vi "parcour_fahren.vi"() -> ()   [LabVIEW 2019]
uses:
  <vilib>/Analysis/_algsub.llb/Vector Norm Type.ctl
  <vilib>/Analysis/baseanly.llb/A x Vector.vi
  <vilib>/Analysis/_algsub.llb/Real Vector Norm.vi
  parcour_liste/parcour_Liste.lvclass
  <vilib>/Analysis/NI_AALPro.lvlib
  <vilib>/Analysis/NI_AALBase.lvlib
panel:
  in  "gain Lenkung":dbl=0.5
  in  "Startkoord":dbl[](array[numeric])=[0.0, 0.0, 0.0]
  in  "v":dbl=20.0
  in  "Ts":dbl=0.02
  out "Sensorwert c":dbl format="%_4g"
  out "Position":dbl[](array[numeric])=[13.46599999999989, 0.0, 0.0] format="%_3g"
  out "XY Graph":cluster{"x":dbl[], "y":dbl[]}[](graph)=[{"x"=[0.0, 200.0], "y"=[0.0, 0.0]}, {"x"=[260.0, 259.2613004357083, 257.0633909777092, 253.4603914513021, 248.54101966249686, 242.42640687119285, 235.2671151375484, 227.2394299843728, 218.54101966249684, 209.38606790241386, 200.0], "y"=[60.0, 50.613932097586144, 41.45898033750316, 32.760570015627195, 24.732884862451613, 17.573593128807154, 11.45898033750315, 6.5396085486979345, 2.9366090222907886, 0.7386995642917356, 0.0]}, {"x"=[260.0, 259.5075336238055, 258.04226065180615, 255.64026096753472, 252.3606797749979, 248.2842712474619, 243.51141009169893, 238.15961998958187, 232.3606797749979, 226.25737860160925, 220.0], "y"=[60.0, 66.25737860160923, 72.36067977499789, 78.15961998958187, 83.51141009169893, 88.2842712474619, 92.36067977499789, 95.64026096753472, 98.04226065180615, 99.50753362380551, 100.0]}, {"x"=[0.0, 220.0], "y"=[100.0, 100.0]}, {"x"=[-40.0, -39.507533623805514, -38.04226065180614, -35.640260967534715, -32.3606797749979, -28.284271247461902, -23.511410091698927, -18.159619989581874, -12.360679774997898, -6.257378601609237, -2.4492935982947065e-15], "y"=[60.0, 66.25737860160923, 72.36067977499789, 78.15961998958187, 83.51141009169893, 88.2842712474619, 92.36067977499789, 95.64026096753472, 98.04226065180615, 99.50753362380551, 100.0]}, {"x"=[-40.0, -40.0], "y"=[60.0, 40.0]}, {"x"=[-40.0, -39.507533623805514, -38.04226065180614, -35.640260967534715, -32.3606797749979, -28.284271247461902, -23.511410091698927, -18.159619989581874, -12.360679774997898, -6.257378601609237, -2.4492935982947065e-15], "y"=[40.0, 33.74262139839077, 27.639320225002102, 21.84038001041813, 16.488589908301073, 11.715728752538102, 7.639320225002102, 4.359739032465285, 1.9577393481938614, 0.49246637619448563, 0.0]}, {"x"=[13.46599999999989, 35.46599999999989, 35.46599999999989, 13.46599999999989, 13.46599999999989], "y"=[7.0, 7.0, -7.0, -7.0, 7.0]}, {"x"=[10.46599999999989, 16.465999999999887, 16.465999999999887, 10.46599999999989, 10.46599999999989], "y"=[8.5, 8.5, 7.5, 7.5, 8.5]}, {"x"=[10.46599999999989, 16.465999999999887, 16.465999999999887, 10.46599999999989, 10.46599999999989], "y"=[-7.5, -7.5, -8.5, -8.5, -7.5]}, {"x"=[32.46599999999989, 38.46599999999989, 38.46599999999989, 32.46599999999989, 32.46599999999989], "y"=[8.5, 8.5, 7.5, 7.5, 8.5]}, {"x"=[32.46599999999989, 38.46599999999989, 38.46599999999989, 32.46599999999989, 32.46599999999989], "y"=[-7.5, -7.5, -8.5, -8.5, -7.5]}, {"x"=[36.46599999999989, 36.46599999999989, 36.46599999999989, 36.46599999999989, 36.46599999999989], "y"=[6.0, 0.0, -6.0, -6.0, -6.0]}]
  out "Lenkwinkel [rad]":dbl
  in  "stop":bool
  in  "milliseconds to wait":u32=10
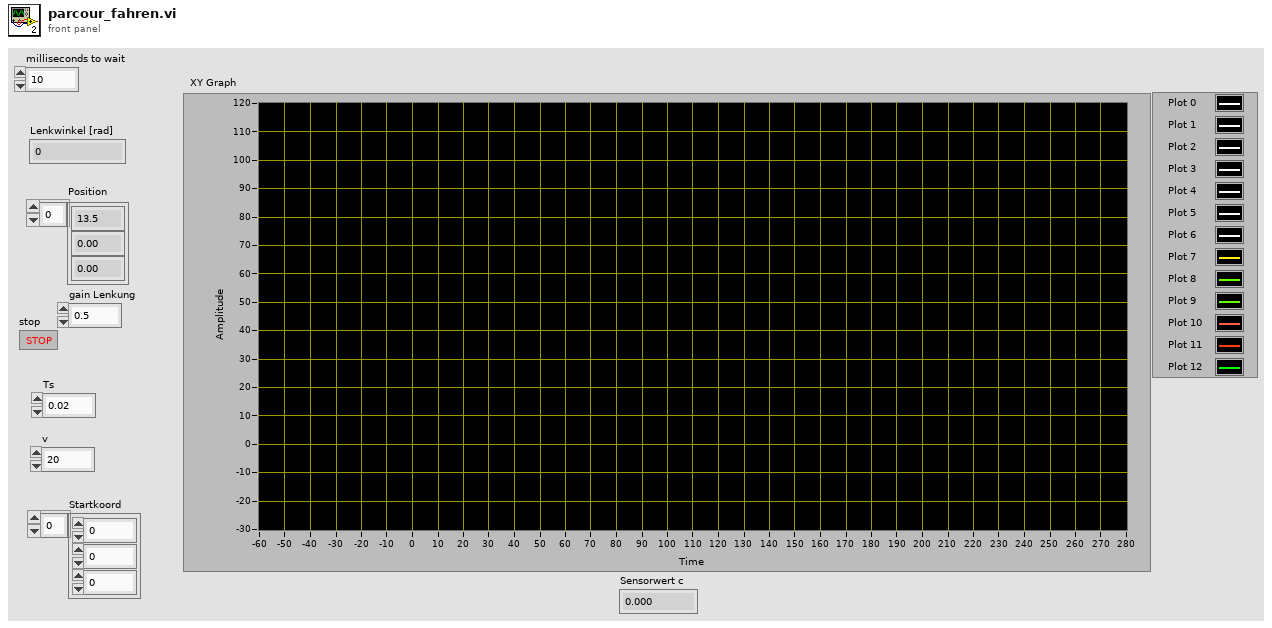
[diagram p1: front panel]
types:
  T1 = typedef "NI_Matrix.lvlib/RealMatrix.ctl" = dbl[][]
  T2 = typedef "NI_AALPro.lvlib/Vector Norm Type.ctl" = u16
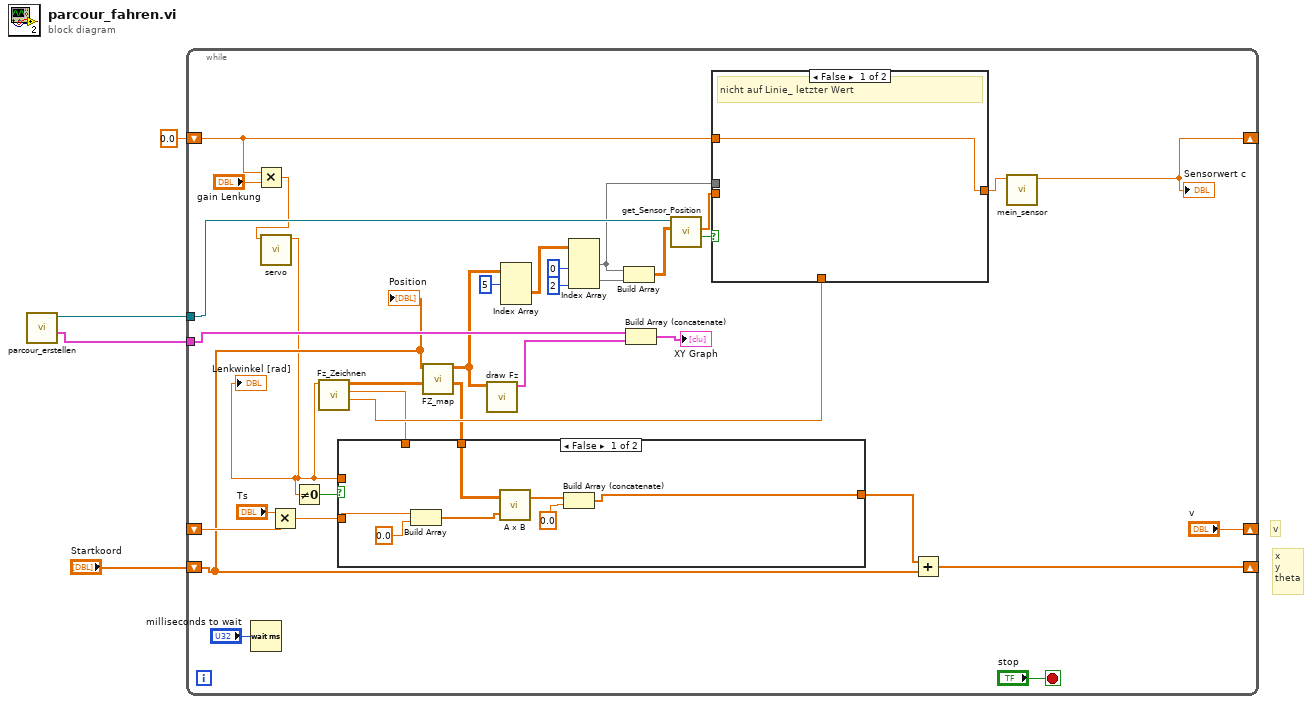
[diagram p0: block diagram]
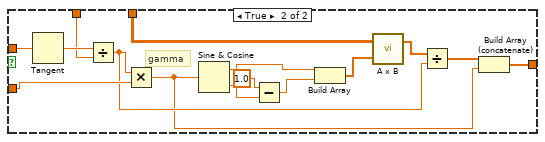
[diagram p2: hidden frame]
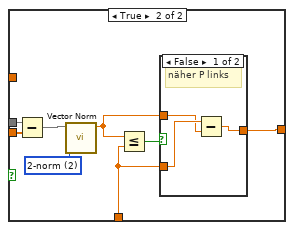
[diagram p3: hidden frame]
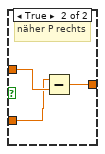
[diagram p4: hidden frame]
diagram:
  # "x\ny\ntheta"
  # "v"
  n1 = call "parcour_erstellen.vi"() -> ("XY_Parcout"=w3:cluster{"x":dbl[], "y":dbl[]}[], "parcour_Liste out"=w4:refnum<class "parcour_Liste.lvclass">)  [unwired: 10 in]
  n2 = while {
    tunnel: w4 -> [w25]
    tunnel: w3 -> [w36]
    shift-right: [w5] -> _
    shift-left: 0.0 -> [w9]
    shift-right: ["v"] -> _
    shift-left: _ -> [w16]
    shift-right: [w12] -> _
    shift-left: "Startkoord" -> [w11]
    stop <- "stop" stop-if-true
    n3 = Wait (ms)(milliseconds to wait="milliseconds to wait") -> ()  [unwired: 1 out]
    n4 = Multiply(x=w9, y="gain Lenkung") -> (x*y=w7:dbl)
    n5 = call "servo.vi"("Winkel soll"=w7) -> ("Winkel ist"=w6:dbl)  [unwired: 10 in]
    "Lenkwinkel [rad]" <- w6
    n6 = Multiply(x="Ts", y=w16) -> (x*y=w15:dbl)
    n7 = Not Equal To 0?(x=w6) -> (x != 0?=w10:bool)
    n8 = call "Fz_Zeichnen.vi"("Lenkwinkel [rad]"=w6) -> ("Breite Sensor/2 [cm] out"=w22:dbl, "Achsabstand [cm] out"=w18:dbl, "Fz"=w35:dbl[][][])  [unwired: 8 in]
    n9 = call "FZ_map.vi"("Fz"=w35, "Position"=w11) -> ("Rot(theta)"=w14:dbl[][], "FZ-mapped"=w32:dbl[][][])  [unwired: 8 in]
    n10 = case shown="False" w10 {
      tunnel: w6 -> [_ w60]
      tunnel: w18 -> [_ w58]
      tunnel: w15 -> [w45 w57]
      tunnel: w14 -> [w43 w51]
      tunnel: [w39 w46] -> w13
      frame False {
        n11 = Build Array(w45, 0.0 ("element")) -> (w42:dbl[])
        n12 = call-poly <vilib>:"A x B.vi"("Vector"=w42, "A"=w43) -> ("A x Vector"=w41:dbl[])  [unwired: 1 out]
        n13 = Build Array (concatenate)(w41, 0.0 ("element")) -> (w39:dbl[])
      }
      frame True {
        # "gamma"
        n14 = Tangent(1:w60) -> (0:w59:dbl)
        n15 = Divide(x=w59, y=w58) -> (x/y=w49:dbl)
        n16 = Multiply(x=w49, y=w57) -> (x*y=w47:dbl)
        n17 = Sine & Cosine(0:w47) -> (1:w53:dbl, 2:w56:dbl)
        n18 = Subtract(x=1.0, y=w56) -> (x-y=w54:dbl)
        n19 = Build Array(w53, w54) -> (w52:dbl[])
        n20 = call-poly <vilib>:"A x B.vi"("Vector"=w52, "A"=w51) -> ("A x Vector"=w50:dbl[])  [unwired: 1 out]
        n21 = Divide(x=w50, y=w49) -> (x/y=w48:dbl[])
        n22 = Build Array (concatenate)(w48, w47) -> (w46:dbl[])
      }
    }
    n23 = call "draw Fz.vi"("FZ"=w32) -> ("X_Y_Plot"=w34:cluster{"x":dbl[], "y":dbl[]}[])  [unwired: 10 in]
    n24 = Index Array(array=w32, index (dim 0)=5 ("index (page)")) -> (element=w30:dbl[][])  [unwired: 2 in]
    n25 = Index Array(array=w30, index (col) #1=0 ("disabled index (col)"), index (col) #2=2 ("index (col)")) -> (element #1=w24:dbl[], element #2=w27:dbl[])  [unwired: 2 in]
    n26 = Build Array(w24, w27) -> (w26:T1)
    n27 = Build Array (concatenate)(w36, w34) -> (→"XY Graph":cluster{"x":dbl[], "y":dbl[]}[])
    n28 = call "get_Sensor_Position.vi"("Sensorkoord [P1 P2]"=w26, "parcour_Liste in"=w25) -> ("Sensor auf Linie"=w21:bool, "Schnittpunkt"=w23:dbl[])  [unwired: 6 in, 2 out]
    n29 = case shown="False" w21 {
      tunnel: w24 -> [_ w68]
      tunnel: w23 -> [_ w67]
      tunnel: w22 -> [_ w63]
      tunnel: [w61 w62] -> w20
      tunnel: w9 -> [w61 _]
      frame False {
        # "nicht auf Linie_ letzter Wert"
      }
      frame True {
        w69 = T2 2 items=["1-norm"=1, "2-norm"=2, "Inf-norm"=3, "-Inf-norm"=4, "User Defined"=5] ("norm type")
        n30 = Subtract(x=w68, y=w67) -> (x-y=w66:dbl[])
        n31 = call-poly <vilib>:"Vector Norm.vi"("norm type"=w69, "Input Vector"=w66) -> ("norm"=w64:dbl)  [unwired: 8 in, 1 out]
        n32 = Less Or Equal?(x=w64, y=w63) -> (x <= y?=w65:bool)
        n33 = case shown="False" w65 {
          tunnel: w64 -> [w71 w75]
          tunnel: w63 -> [w72 w74]
          tunnel: [w70 w73] -> w62
          frame False {
            # "näher P links"
            n34 = Subtract(x=w72, y=w71) -> (x-y=w70:dbl)
          }
          frame True {
            # "näher P rechts"
            n35 = Subtract(x=w74, y=w75) -> (x-y=w73:dbl)
          }
        }
      }
    }
    n36 = Add(x=w13, y=w11) -> (x+y=w12:dbl[])
    n37 = call "mein_sensor.vi"("Position"=w20) -> ("Sensorsignal"=w5:dbl)  [unwired: 10 in]
    "Sensorwert c" <- w5
    "Position" <- w11
  }
